vi "Configure Table Operation.vi"(8 "New Table Name (\"MyTable\")":string="MyTable", 9 "Table Name (\"DEFAULT\")":string="DEFAULT", 10 "Table Data":i32[](array[numeric]), 11 "Operation (1: Define Frequency Array)":i32(ring)=1 items=["Define Frequency Array"=1, "Rename Existing Table"=3, "Clear Existing Table"=4]) -> (1 "ResultString":string)   [LabVIEW 2018, in "Agilent U2000 Series.lvlib"]
doc: "Operates instrument for table functionality. Includes: Defines frequency array, renames or clears specified table."
uses:
  Agilent U2000 Series.lvlib
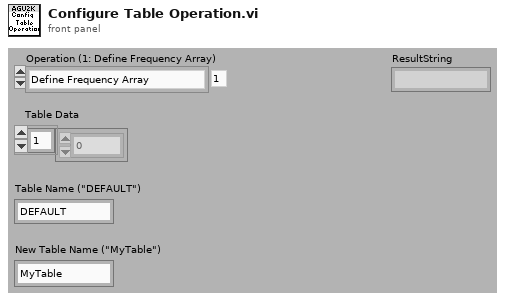
[diagram p1: front panel]
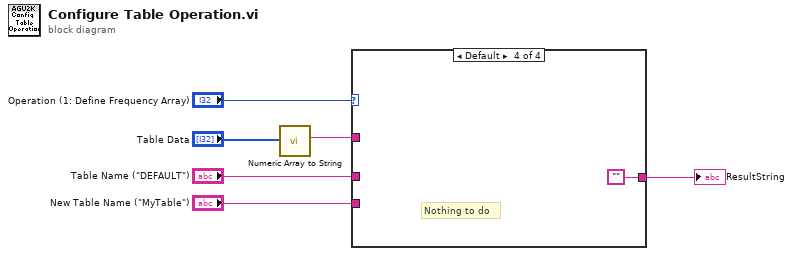
[diagram p0: block diagram]
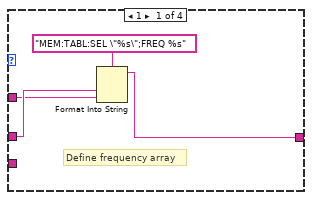
[diagram p2: hidden frame]
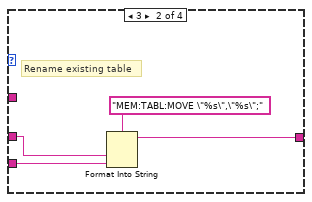
[diagram p3: hidden frame]
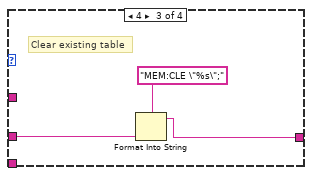
[diagram p4: hidden frame]
diagram:
  n1 = call "Numeric Array to String.vi"("List Data"="Table Data") -> ("Result String"=w3:string)  [unwired: 10 out]
  n2 = case shown="Default" "Operation (1: Define Frequency Array)" {
    tunnel: w3 -> [w8 _ _ _]
    tunnel: "Table Name (\"DEFAULT\")" -> [w9 w13 w15 _]
    tunnel: "New Table Name (\"MyTable\")" -> [_ w12 _ _]
    tunnel: [w7 w11 w16 ""] -> w6
    frame 1 {
      # "Define frequency array"
      n3 = Format Into String(format string="MEM:TABL:SEL \"%s\";FREQ %s", w9, w8) -> (resulting string=w7:string)  [unwired: 2 in, 1 out]
    }
    frame 3 {
      # "Rename existing table"
      n4 = Format Into String(format string="MEM:TABL:MOVE \"%s\",\"%s\";", w13, w12) -> (resulting string=w11:string)  [unwired: 2 in, 1 out]
    }
    frame 4 {
      # "Clear existing table"
      n5 = Format Into String(format string="MEM:CLE \"%s\";", w15) -> (resulting string=w16:string)  [unwired: 2 in, 1 out]
    }
    frame Default {
      # "Nothing to do"
    }
  }
  "ResultString" <- w6
